vi "kvCanGetBusParams.vi"(2 "Channel Handle (input only)":i32, 3 "error in (no error)":errorcluster) -> (0 "CAN Bus Frequency":u32, 1 "Time Segment 1":u32, 4 "Synchronization Jump Width":u32, 5 "Time Segment 2":u32, 6 "error out":errorcluster, 7 "Channel Handle (ouput only)":i32, 8 "Number of Sampling Points":u32, 9 "Sync Mode":u32)   [LabVIEW 2022 SP3]
doc: "This function retrieves the current bus parameters for the specified channel."
uses:
  canlib32.dll
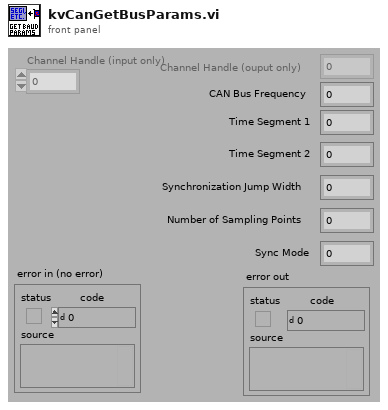
[diagram p1: front panel]
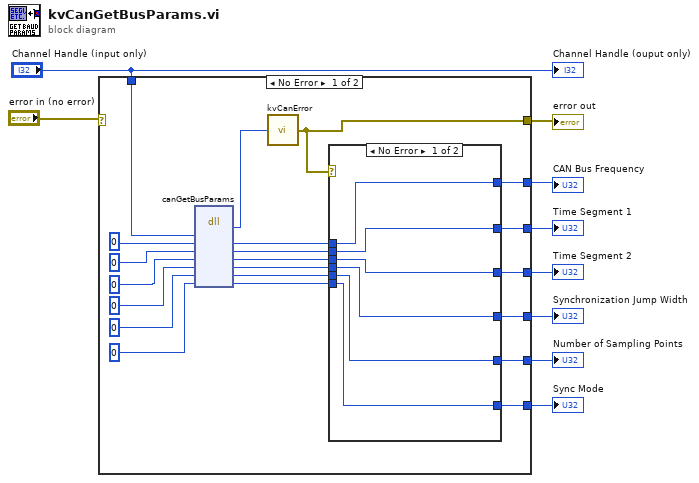
[diagram p0: block diagram]
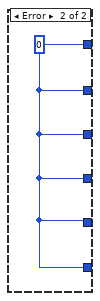
[diagram p2: hidden frame]
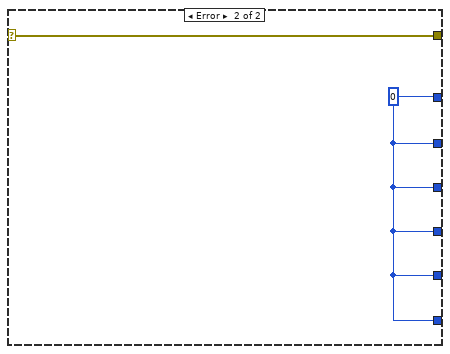
[diagram p3: hidden frame]
diagram:
  n1 = case shown="No Error" "error in (no error)" {
    selector: "error in (no error)" -> [_ w39]
    tunnel: [w23 w39] -> w8
    tunnel: "Channel Handle (input only)" -> [w24 _]
    tunnel: [w22 w38] -> w6
    tunnel: [w20 w38] -> w5
    tunnel: [w18 w38] -> w4
    tunnel: [w16 w38] -> w3
    tunnel: [w13 w38] -> w2
    tunnel: [w11 w38] -> w1
    frame No Error {
      n2 = dll-call lib="canlib32.dll" fn="canGetBusParams"("handle"=w24, "freq"=0, "tseg1"=0, "tseg2"=0, "sjw"=0, "nosamp"=0, "syncmode"=0) -> (w25:i32, "freq"=w21:i32, "tseg1"=w19:u32, "tseg2"=w17:u32, "sjw"=w15:u32, "nosamp"=w14:u32, "syncmode"=w12:u32)  [unwired: 4 in, 2 out]
      n3 = call "kvCanError.vi"("error code"=w25) -> ("error out"=w23:errorcluster)
      n4 = case shown="No Error" w23 {
        tunnel: [w36 w37] -> w22
        tunnel: w21 -> [w36 _]
        tunnel: [w35 w37] -> w20
        tunnel: w19 -> [w35 _]
        tunnel: [w34 w37] -> w18
        tunnel: w17 -> [w34 _]
        tunnel: [w33 w37] -> w16
        tunnel: w15 -> [w33 _]
        tunnel: w14 -> [w31 _]
        tunnel: [w32 w37] -> w13
        tunnel: w12 -> [w32 _]
        tunnel: [w31 w37] -> w11
        frame No Error {
        }
        frame Error {
          w37 = 0
        }
      }
    }
    frame Error {
      w38 = 0
    }
  }
  "Time Segment 1" <- w5
  "Time Segment 2" <- w4
  "Synchronization Jump Width" <- w3
  "Number of Sampling Points" <- w1
  "Sync Mode" <- w2
  "error out" <- w8
  "CAN Bus Frequency" <- w6
  "Channel Handle (ouput only)" <- "Channel Handle (input only)"
